vi "缓冲字符串.vi"(6 "分隔符 (\"\")":string, 9 "缓冲长度":u8=15, 11 "添加新字符串":string) -> (3 "缓冲字符串":string)   [LabVIEW 2012]
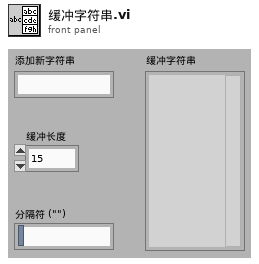
[diagram p1: front panel]
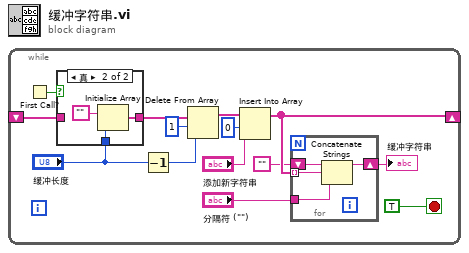
[diagram p0: block diagram]
diagram:
  n1 = while {
    shift-right: [w6] -> _
    shift-left: _ -> [w13]
    stop <- TRUE stop-if-true
    n2 = First Call?() -> (First Call?: T/F=w14:bool)
    n3 = case shown="真" w14 {
      tunnel: [w19 w21] -> w12
      tunnel: w13 -> [w19 _]
      tunnel: "缓冲长度" -> [_ w20]
      frame False {
      }
      frame True {
        n4 = Initialize Array("" ("element"), w20) -> (w21:string[])
      }
    }
    n5 = Decrement(x="缓冲长度") -> (x-1=w10:u8)
    n6 = Delete From Array(array=w12, length=1, index=w10) -> (array with subset deleted=w8:string[])  [unwired: 1 out]
    n7 = Insert Into Array(array=w8, index=0, new element="添加新字符串") -> (w6:string[])
    n8 = for {
      tunnel: w6 -> [w17] mode=indexing
      shift-right: [w16] -> w4
      shift-left: "" ("element") -> [w18]
      tunnel: "分隔符 (\"\")" -> [w15]
      n9 = Concatenate Strings(w18, w17, w15) -> (w16:string)
    }
    "缓冲字符串" <- w4
  }
